vi "acquireIndexClosetoCertainFrequency.vi"(1 "input_array_freDemand":string[](array[string]), 2 "input_array_freArray":string[](array[string])) -> (0 "show_array_index":dbl[](array[numeric]))   [LabVIEW 2011]
panel:
  out "数字 2":dbl[](array[numeric])
  out "数字":dbl[](array[numeric])
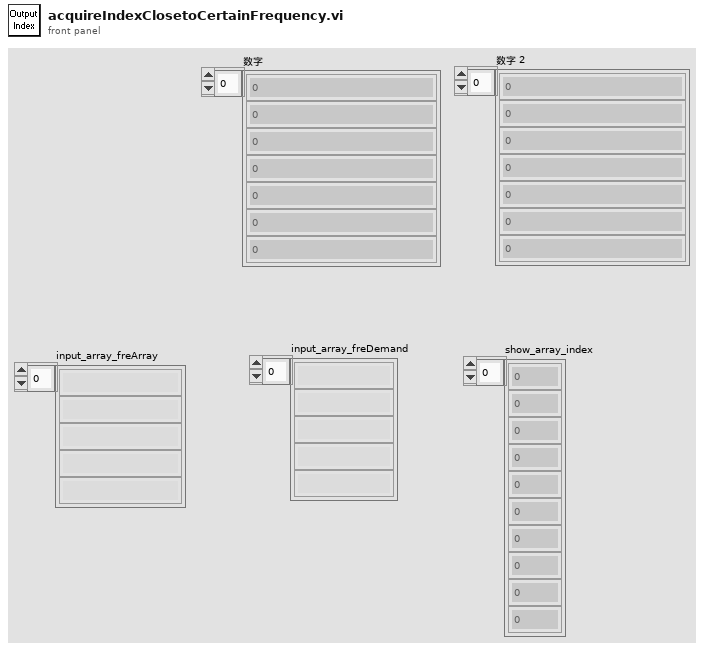
[diagram p1: front panel]
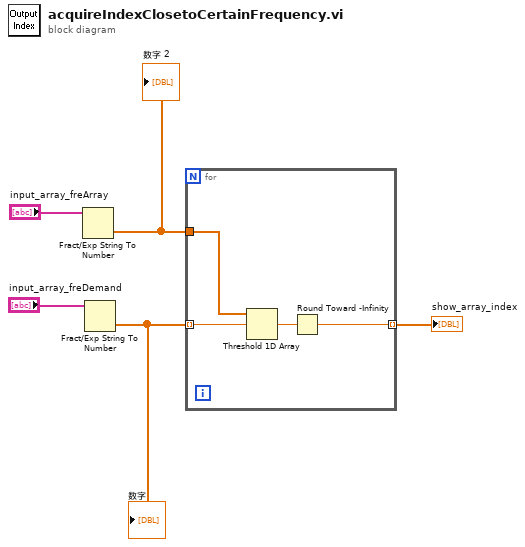
[diagram p0: block diagram]
diagram:
  n1 = Fract/Exp String To Number(string="input_array_freArray") -> (number=w3:dbl[])  [unwired: 3 in, 1 out]
  "数字 2" <- w3
  n2 = Fract/Exp String To Number(string="input_array_freDemand") -> (number=w1:dbl[])  [unwired: 3 in, 1 out]
  "数字" <- w1
  n3 = for {
    tunnel: w1 -> [w9] mode=indexing
    tunnel: w3 -> [w8]
    tunnel: [w6] -> w2 mode=indexing
    n4 = Threshold 1D Array(2:w9, 3:w8) -> (0:w7:dbl)  [unwired: 1 in]
    n5 = Round Toward -Infinity(1:w7) -> (0:w6:dbl)
  }
  "show_array_index" <- w2
